vi "FGV Messwerte_FID.vi"(0 "GasValue":sgl[](array[numeric]), 1 "Messbereich":T3 items=["0-500ppm"=1, "0-2500ppm"=2, "0-10000ppm"=3], 4 "Zielmessbereich":u16, 7 "Prüfgaskonz.":sgl, 8 "Kalibrieren":T1, 9 "Aktion":T5=enum."Messen", 13 "CAL-Daten Tolernaz":T2) -> (14 "Rohwert LIN":sgl[](array[numeric]), 16 "Rohwerte":sgl[](array[numeric]), 19 "im gültigen Bereich":bool, 20 "GasValue":sgl[](array[numeric]), 21 "CAL-Daten":T4={"CH4 Null"=0.0, "CH4 Steil"=[1.0, 1.0, 1.0, 1.0], "THC Null"=0.0, "THC Steil"=[1.0, 1.0, 1.0, 1.0], "NMHC Null"=0.0, "NMHC Steil"=[1.0, 1.0, 1.0, 1.0]}, 24 "CAL-Daten Tolernaz":T2, 25 "Kalibrieren erfolgreich":bool, 27 "CAL TimeOut":bool)   [LabVIEW 2020, in "ABB-EL3000.lvlib" / "FID.lvlib" / "FID Kalibrierung.lvlib"]
uses:
  FID Kalibrierung.lvlib
  Allgemeine VI/FGV Uras26 Aktion.ctl
  Allgemeine VI/CAL-Daten FID.ctl
  Allgemeine VI/Messbereich CO lo.ctl
  Allgemeine VI/CAL-Daten Toleranz.ctl
  FID Kalibrieren.ctl
  Auto Kalibrieren/KAL Daten loggen Aktionen.ctl
  Allgemeine VI/Aktionen Cal Daten speichern.ctl
  Allgemein/allgemeine Sub-VIs.lvlib
  Allgemeine VI/Allgemeine VI.lvlib
  Auto Kalibrieren/Auto Kalibrieren.lvlib
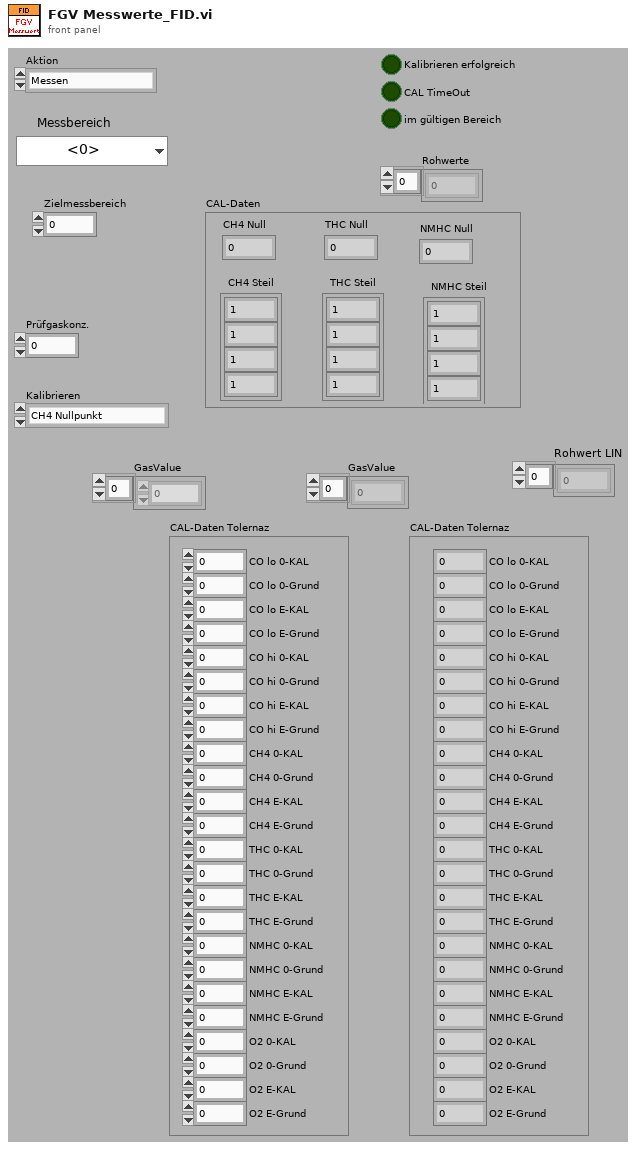
[diagram p1: front panel]
types:
  T1 = typedef "ABB-EL3000.lvlib/FID.lvlib/FID Kalibrierung.lvlib/FID Kalibrieren.ctl" = enum16{"CH4 Nullpunkt", "THC Nullpunkt", "NMHC Nullpunkt", "CH4 Endpunkt", "THC Endpunkt", "NMHC Endpunkt"}
  T2 = typedef "ABB-EL3000.lvlib/Allgemeine VI.lvlib/CAL-Daten Toleranz.ctl" = cluster{"CO lo 0-KAL":sgl, "CO lo 0-Grund":sgl, "CO lo E-KAL":sgl, "CO lo E-Grund":sgl, "CO hi 0-KAL":sgl, "CO hi 0-Grund":sgl, "CO hi E-KAL":sgl, "CO hi E-Grund":sgl, "CH4 0-KAL":sgl, "CH4 0-Grund":sgl, "CH4 E-KAL":sgl, "CH4 E-Grund":sgl, "THC 0-KAL":sgl, "THC 0-Grund":sgl, "THC E-KAL":sgl, "THC E-Grund":sgl, "NMHC 0-KAL":sgl, "NMHC 0-Grund":sgl, "NMHC E-KAL":sgl, "NMHC E-Grund":sgl, "O2 0-KAL":sgl, "O2 0-Grund":sgl, "O2 E-KAL":sgl, "O2 E-Grund":sgl}
  T3 = typedef "ABB-EL3000.lvlib/Allgemeine VI.lvlib/Messbereich CO lo.ctl" = u16
  T4 = typedef "ABB-EL3000.lvlib/Allgemeine VI.lvlib/CAL-Daten FID.ctl" = cluster{"CH4 Null":sgl, "CH4 Steil":sgl[], "THC Null":sgl, "THC Steil":sgl[], "NMHC Null":sgl, "NMHC Steil":sgl[]}
  T5 = typedef "ABB-EL3000.lvlib/Allgemeine VI.lvlib/FGV Uras26 Aktion.ctl" = enum16{"lesen", "CAL-Daten laden", "Messen", "Kalibrieren vorbereiten", "Kalibrieren", "CAL-Daten speichern", "Toleranz schreiben", "CAL-Daten kopieren"}
  T6 = typedef "Auto Kalibrieren.lvlib/KAL Daten loggen Aktionen.ctl" = enum16{"lesen", "initialisieren", "loggen"}
  T7 = typedef "ABB-EL3000.lvlib/Allgemeine VI.lvlib/Aktionen Cal Daten speichern.ctl" = enum16{"Cal Daten", "Toleranzen", "PMA", "FID", "Cal Daten PMA", "Cal Daten FID"}
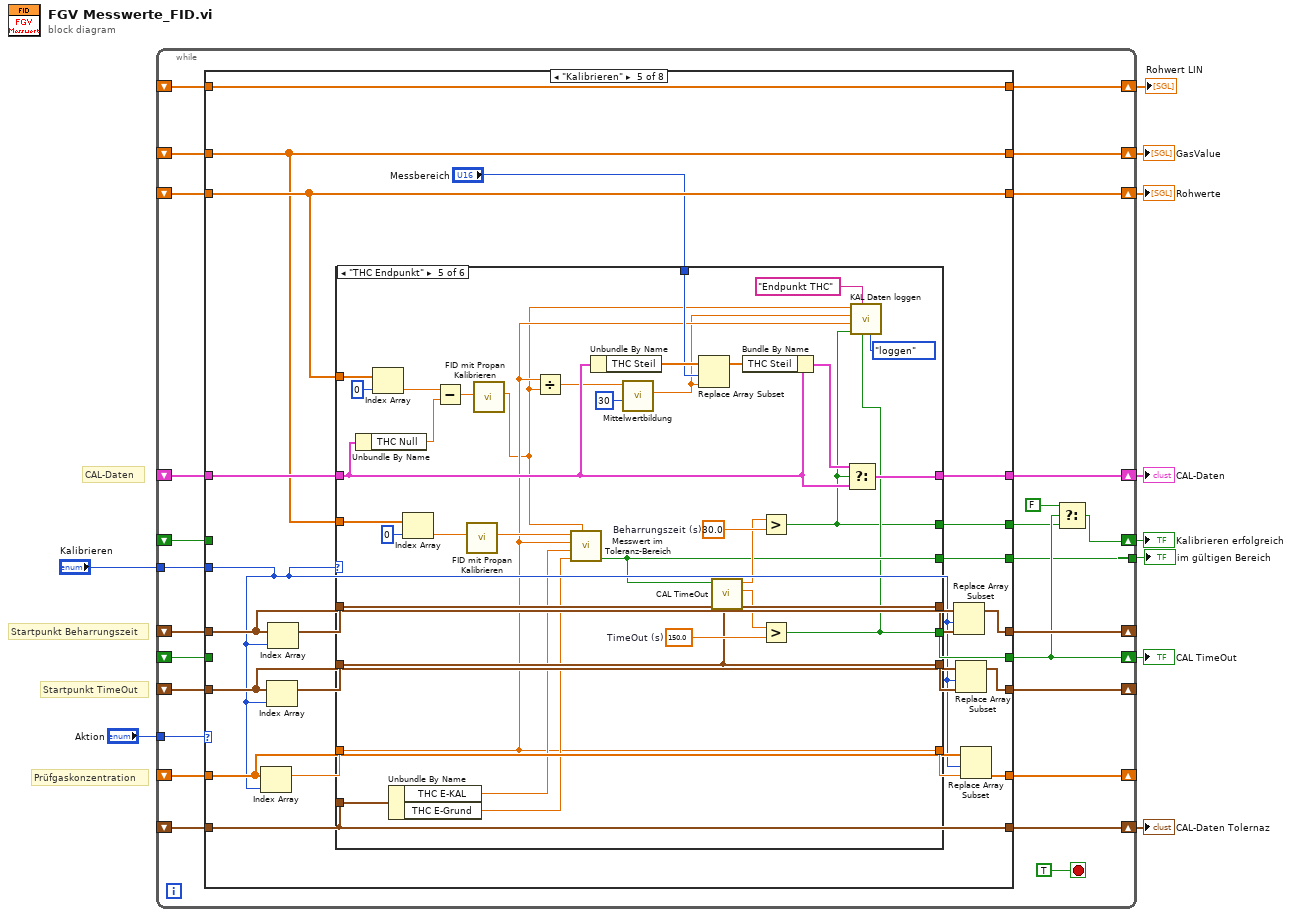
[diagram p0: block diagram]
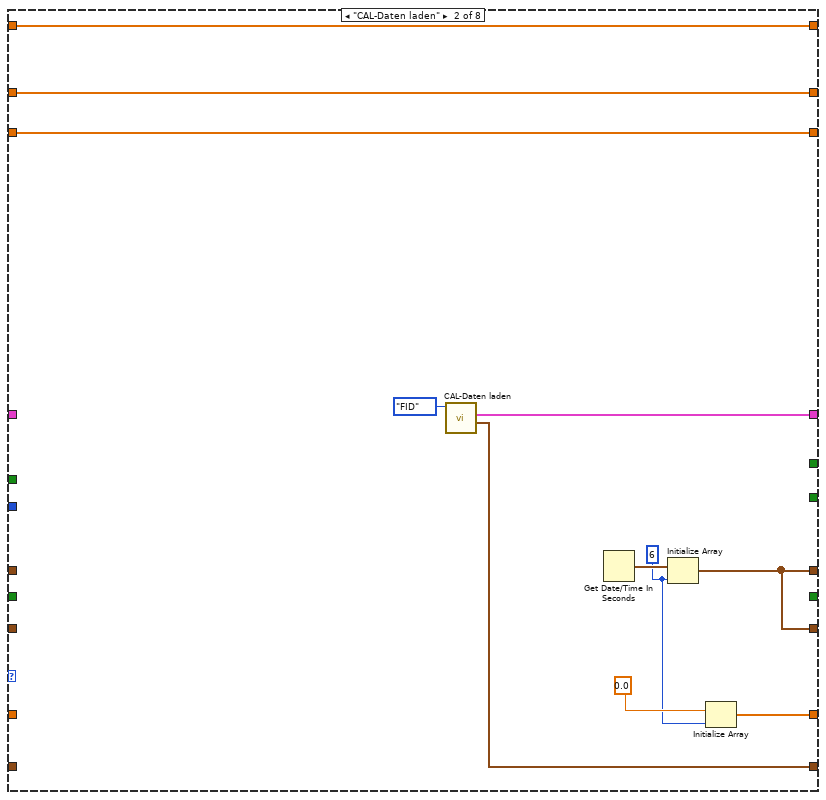
[diagram p3: hidden frame]
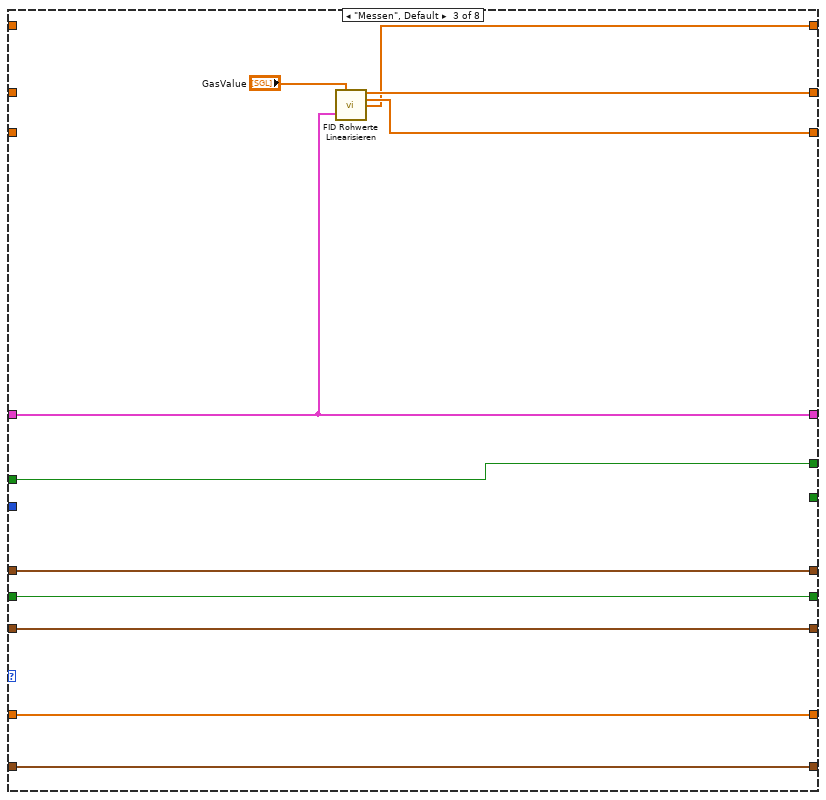
[diagram p4: hidden frame]
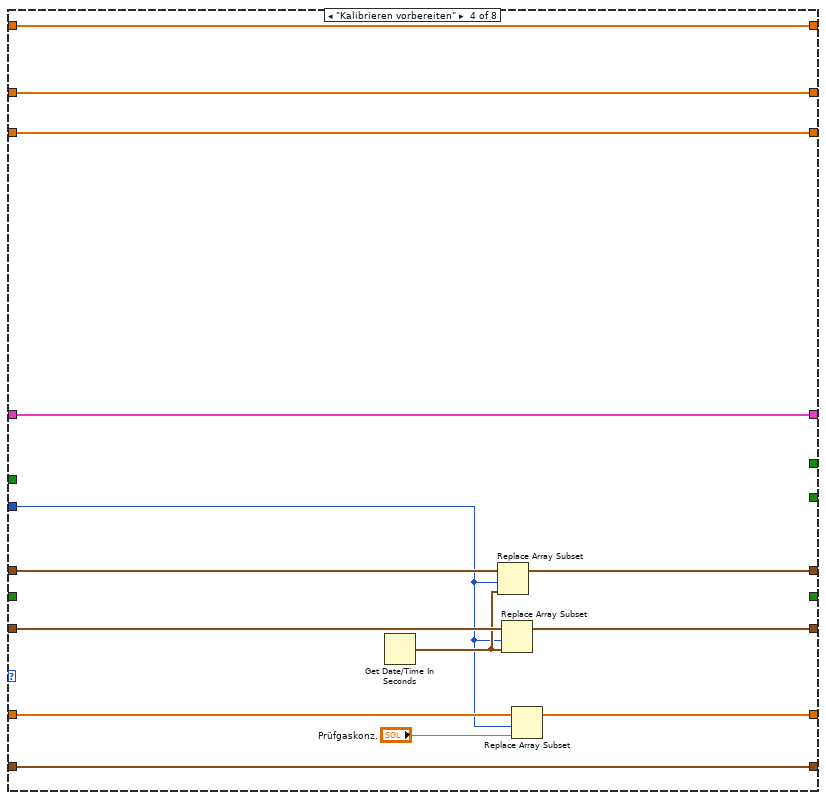
[diagram p5: hidden frame]
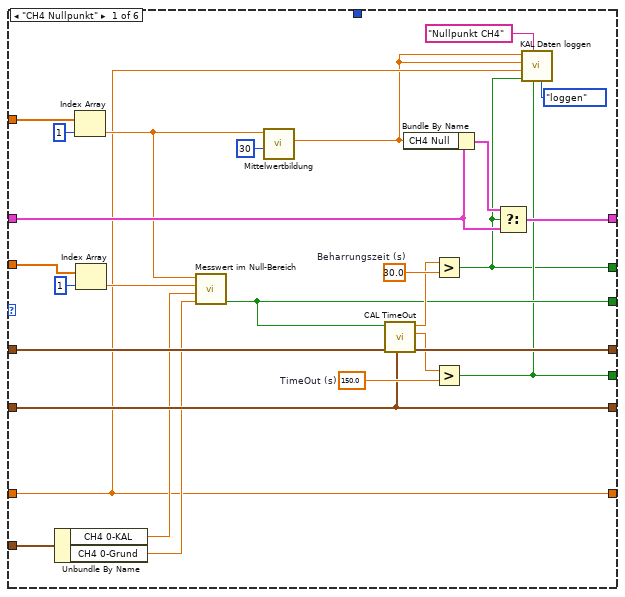
[diagram p6: hidden frame]
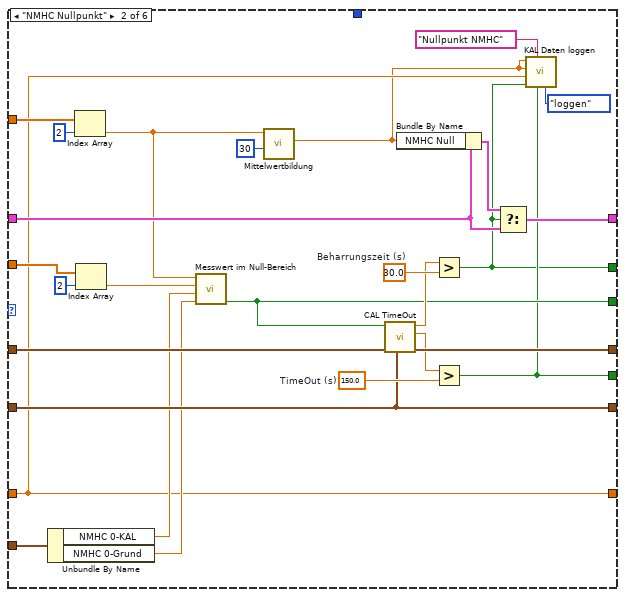
[diagram p7: hidden frame]
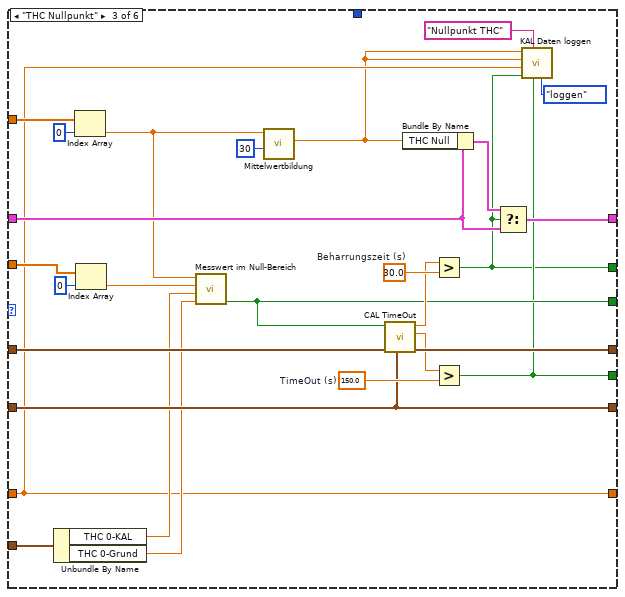
[diagram p8: hidden frame]
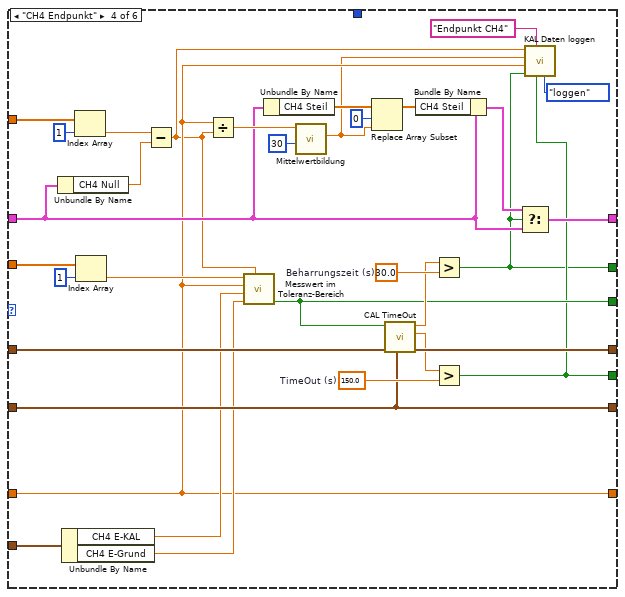
[diagram p9: hidden frame]
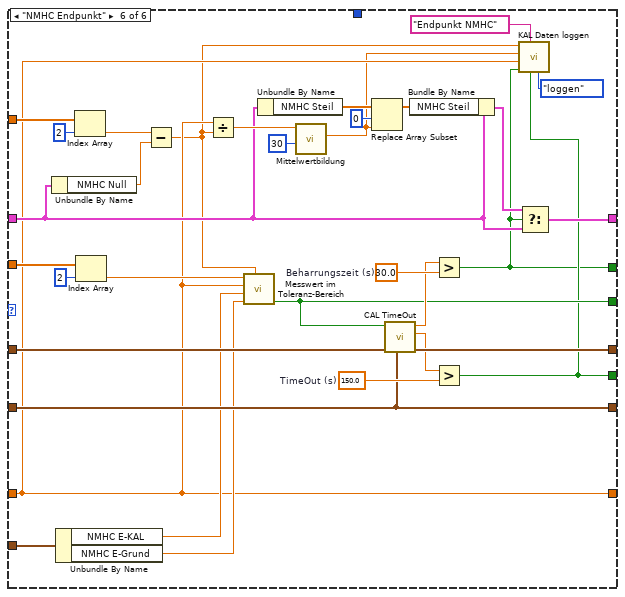
[diagram p10: hidden frame]
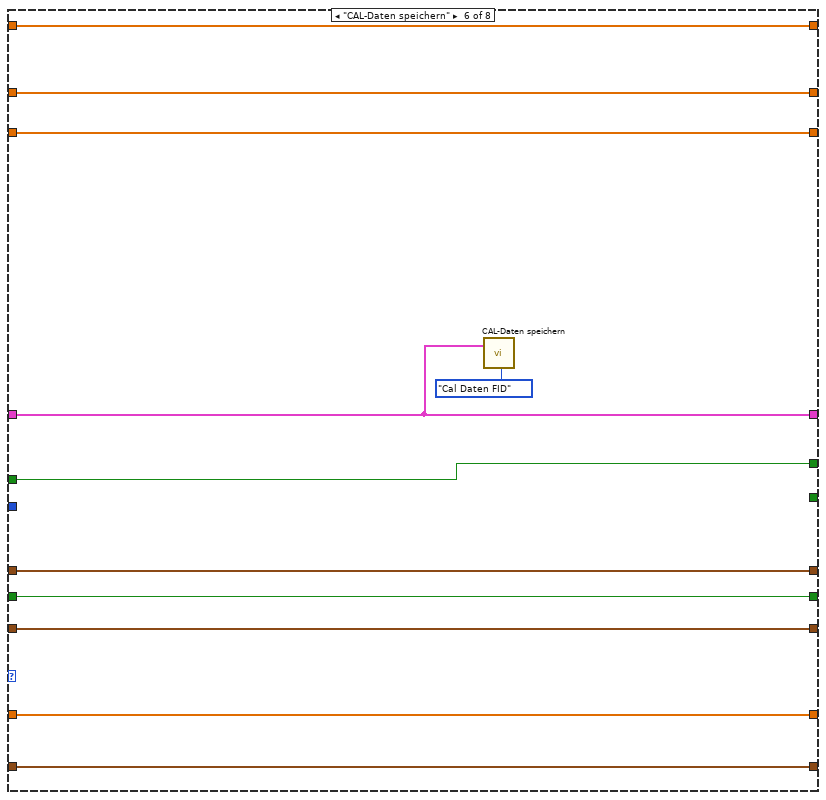
[diagram p11: hidden frame]
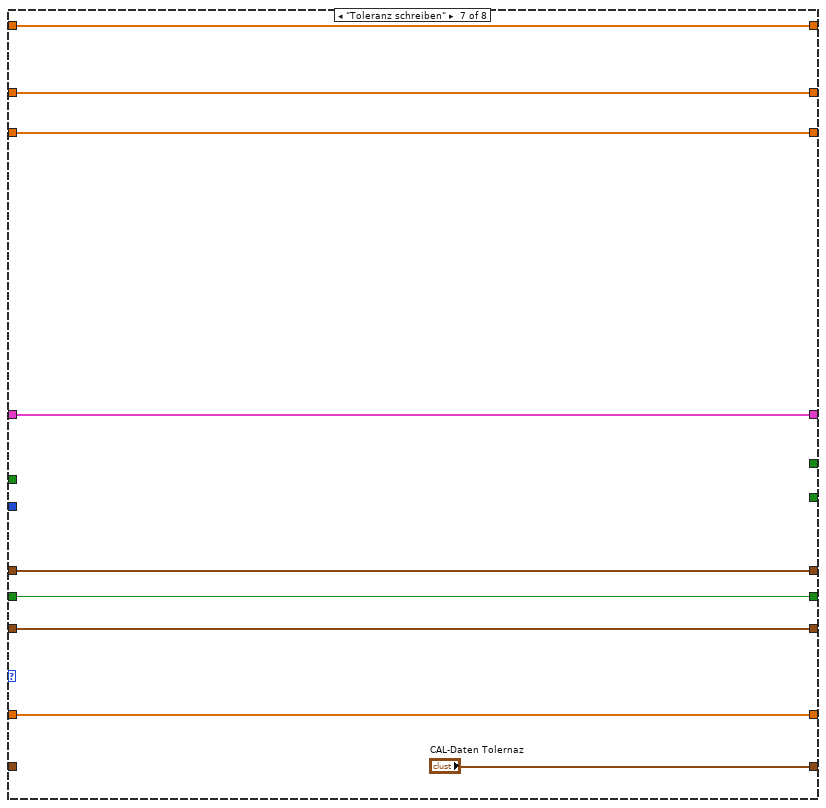
[diagram p12: hidden frame]
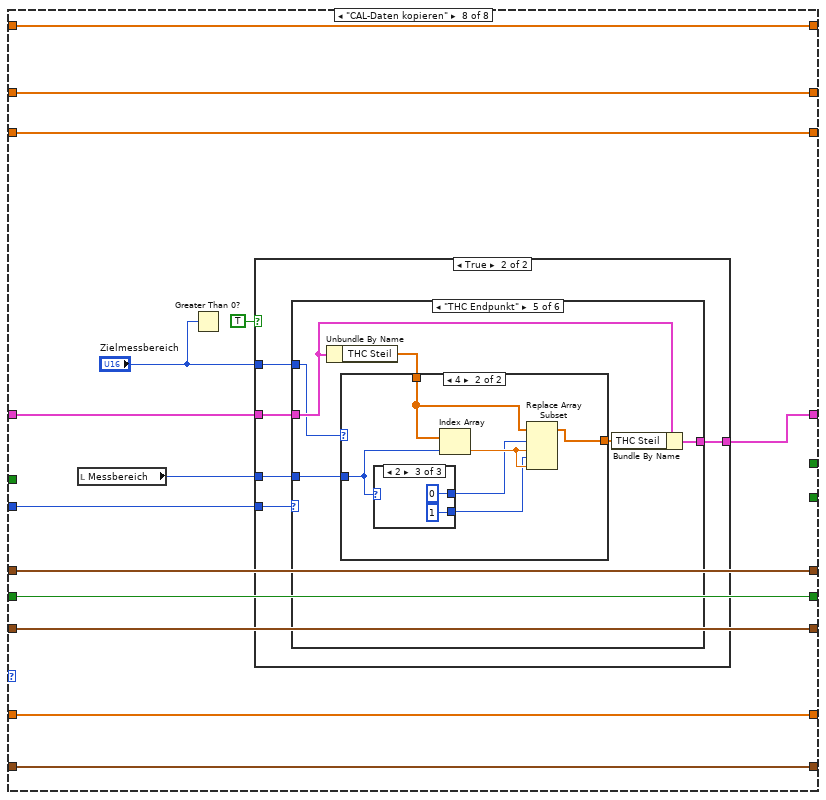
[diagram p13: hidden frame]
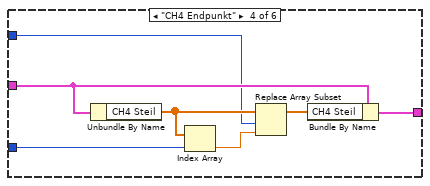
[diagram p18: hidden frame]
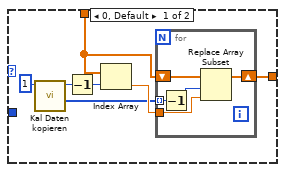
[diagram p19: hidden frame]
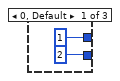
[diagram p20: hidden frame]
diagram:
  # "Prüfgaskonzentration"
  # "Startpunkt TimeOut"
  # "Startpunkt Beharrungszeit"
  # "CAL-Daten"
  n1 = while {
    tunnel: "Aktion" -> [w28]
    shift-right: [w35] -> w7
    shift-left: _ -> [w27]
    tunnel: "Kalibrieren" -> [w34]
    shift-right: [w32] -> _
    shift-left: _ -> [w31]
    shift-right: [w30] -> _
    shift-left: _ -> [w29]
    shift-right: [w22] -> w6
    shift-left: _ -> [w21]
    shift-right: [w24] -> w8
    shift-left: _ -> [w19]
    shift-right: [w26] -> w9
    shift-left: _ -> [w20]
    shift-right: [w18] -> _
    shift-left: _ -> [w33]
    shift-right: [w17] -> w5
    shift-left: _ -> [w16]
    shift-right: [w15] -> w4
    shift-left: _ -> [w14]
    tunnel: [w13] -> w3
    shift-right: [w12] -> w1
    shift-left: _ -> [w11]
    stop <- TRUE stop-if-true
    n2 = case shown="\"Kalibrieren\"" w28 {
      tunnel: w27 -> [w44 _ w62 w80 w101 w288 w304 w317]
      tunnel: [w44 w47 w62 w80 w104 w288 w304 w316] -> w35
      tunnel: w34 -> [_ _ _ w71 w84 _ _ w318]
      tunnel: w33 -> [w41 _ w63 w73 w85 w294 w301 w312]
      tunnel: [w43 w51 w67 w70 w94 w292 w303 w315] -> w32
      tunnel: w31 -> [w43 _ w67 w77 w93 w292 w303 w315]
      tunnel: [w42 w51 w66 w69 w90 w291 w302 w313] -> w30
      tunnel: w29 -> [w42 _ w66 w76 w88 w291 w302 w313]
      tunnel: [_ _ w64 _ w103 w296 w299 w314] -> w26
      tunnel: [w38 _ w65 _ w102 w295 _ _] -> w25
      tunnel: [w45 w56 w58 w81 w99 w297 w305 w319] -> w22
      tunnel: w21 -> [w45 w56 _ w81 w99 w297 w305 w319]
      tunnel: w20 -> [_ _ w64 _ _ w296 w299 w314]
      tunnel: w19 -> [w38 _ w65 _ _ w295 _ _]
      tunnel: [w41 w48 w63 w72 w86 w294 w301 w312] -> w18
      tunnel: [w40 w55 w59 w79 w98 w293 w306 w320] -> w17
      tunnel: w16 -> [w40 w55 _ w79 w98 w293 w306 w320]
      tunnel: [w39 w54 w61 w78 w100 w290 "CAL-Daten Tolernaz" w311] -> w15
      tunnel: w14 -> [w39 _ w61 w78 w100 w290 _ w311]
      tunnel: [_ _ _ _ w97 _ _ _] -> w13
      tunnel: [w37 w46 w57 w68 w82 w287 w298 w307] -> w12
      tunnel: w11 -> [w37 w46 _ w68 w82 w287 w298 w307]
      frame "lesen" {
      }
      frame "CAL-Daten laden" {
        w49 = 6 ("Dimension")
        n3 = call "CAL-Daten laden.vi"("Aktion"=enum16{"PMA", "FID"}."FID") -> ("CAL-Daten Tolernaz"=w54:T2, "CAL-Daten FID"=w47:T4)  [unwired: 6 in, 3 out]
        n4 = Get Date/Time In Seconds() -> (seconds since 1Jan1904=w52:timestamp)
        n5 = Initialize Array(w52, w49) -> (w51:timestamp[])
        n6 = Initialize Array(sgl 0.0 ("Prüfgaskonz."), w49) -> (w48:sgl[])
      }
      frame "Messen", Default {
        n7 = call "FID Rohwerte Linearisieren.vi"("GasValue"="GasValue", "CAL-Daten"=w62) -> ("Messwerte"=w59:sgl[], "Rohwert"=w58:sgl[], "Rohwert LIN"=w57:sgl[])  [unwired: 11 in]
      }
      frame "Kalibrieren vorbereiten" {
        n8 = Get Date/Time In Seconds() -> (seconds since 1Jan1904=w75:timestamp)
        n9 = Replace Array Subset(array=w77, new element=w75, index=w71) -> (w70:timestamp[])
        n10 = Replace Array Subset(array=w76, new element=w75, index=w71) -> (w69:timestamp[])
        n11 = Replace Array Subset(array=w73, new element="Prüfgaskonz.", index=w71) -> (w72:sgl[])
      }
      frame "Kalibrieren" {
        n12 = Index Array(array=w85, index=w84) -> (element=w87:sgl)
        n13 = Index Array(array=w88, index=w84) -> (element=w91:timestamp)
        n14 = Index Array(array=w93, index=w84) -> (element=w95:timestamp)
        n15 = case shown="\"THC Endpunkt\"" w84 {
          tunnel: w101 -> [w122 w149 w176 w199 w236 w267]
          tunnel: [w125 w152 w179 w212 w247 w280] -> w104
          tunnel: w87 -> [w106 w133 w160 w188 w221 w257]
          tunnel: w95 -> [w129 w156 w183 w216 w251 w284]
          tunnel: [w127 w154 w181 w214 w249 w282] -> w92
          tunnel: [w128 w155 w182 w215 w250 w283] -> w89
          tunnel: w91 -> [w128 w155 w182 w215 w250 w283]
          tunnel: [w108 w135 w162 w191 w223 w259] -> w103
          tunnel: [w107 w134 w161 w190 w222 w258] -> w102
          tunnel: [w106 w133 w160 w188 w221 w257] -> w96
          tunnel: w100 -> [w120 w147 w174 w206 w242 w274]
          tunnel: w99 -> [w119 w146 w173 w203 w239 w271]
          tunnel: w98 -> [w118 w145 w172 w201 w238 w269]
          tunnel: "Messbereich" -> [_ _ _ _ w226 _]
          tunnel: [w117 w141 w168 w200 w237 w268] -> w97
          frame "CH4 Nullpunkt" {
            w130 = sgl 150.0  # TimeOut (s)
            w131 = sgl 30.0  # Beharrungszeit (s)
            n16 = Unbundle By Name(w120) -> ("CH4 0-KAL"=w114:sgl, "CH4 0-Grund"=w113:sgl)
            n17 = Index Array(array=w119, index=1 ("Index")) -> (element=w116:sgl)
            n18 = Index Array(array=w118, index=1 ("Index")) -> (element=w115:sgl)
            n19 = call "Messwert im Null-Bereich.vi"("Toleranz Grundkalibrierung"=w113, "Toleranz letzte KAL"=w114, "Messwert"=w115, "Rohwert"=w116) -> ("im Bereich"=w117:bool)  [unwired: 7 in]
            n20 = call "Mittelwertbildung.vi"("Anzahl Werte"=u8 30, "Neuer Wert"=w116) -> ("gemittelter Wert"=w105:sgl)  [unwired: 7 in, 2 out]
            n21 = call "CAL TimeOut.vi"("CAL-Start"=w128, "im Bereich seit"=w129, "im Bereich"=w117) -> ("im Bereich seit (Ausgang)"=w127:timestamp, "Sekunden seit CAL-Start"=w126:sgl, "Sekunden im Bereich"=w124:sgl)  [unwired: 5 in]
            n22 = Bundle By Name(cluster=w122, "CH4 Null"=w105) -> (w123:T4)
            n23 = Greater?(x=w124, y=w131) -> (0:w107:bool)
            n24 = Greater?(x=w126, y=w130) -> (0:w108:bool)
            n25 = Select(t=w123, s=w107, f=w122) -> (s? t:f=w125:T4)
            n26 = call "KAL Daten loggen.vi"("Aktionen MFC loggen"=KAL_Daten_loggen_Aktionen."loggen", "TimeOUT"=w108, "Komponente"="Nullpunkt CH4", "Kalibrieren Erfolgreich"=w107, "Prüfgaskonzentration"=w106, "Kalibrierwert"=w105, "Rohwert"=w105) -> ()  [unwired: 4 in, 1 out]
          }
          frame "NMHC Nullpunkt" {
            w157 = sgl 150.0  # TimeOut (s)
            w158 = sgl 30.0  # Beharrungszeit (s)
            n27 = Unbundle By Name(w147) -> ("NMHC 0-KAL"=w143:sgl, "NMHC 0-Grund"=w142:sgl)
            n28 = Index Array(array=w146, index=2 ("Index")) -> (element=w140:sgl)
            n29 = Index Array(array=w145, index=2 ("Index")) -> (element=w144:sgl)
            n30 = call "Messwert im Null-Bereich.vi"("Toleranz Grundkalibrierung"=w142, "Toleranz letzte KAL"=w143, "Messwert"=w144, "Rohwert"=w140) -> ("im Bereich"=w141:bool)  [unwired: 7 in]
            n31 = call "Mittelwertbildung.vi"("Anzahl Werte"=u8 30, "Neuer Wert"=w140) -> ("gemittelter Wert"=w132:sgl)  [unwired: 7 in, 2 out]
            n32 = call "CAL TimeOut.vi"("CAL-Start"=w155, "im Bereich seit"=w156, "im Bereich"=w141) -> ("im Bereich seit (Ausgang)"=w154:timestamp, "Sekunden seit CAL-Start"=w153:sgl, "Sekunden im Bereich"=w151:sgl)  [unwired: 5 in]
            n33 = Bundle By Name(cluster=w149, "NMHC Null"=w132) -> (w150:T4)
            n34 = Greater?(x=w151, y=w158) -> (0:w134:bool)
            n35 = Greater?(x=w153, y=w157) -> (0:w135:bool)
            n36 = Select(t=w150, s=w134, f=w149) -> (s? t:f=w152:T4)
            n37 = call "KAL Daten loggen.vi"("Aktionen MFC loggen"=KAL_Daten_loggen_Aktionen."loggen", "TimeOUT"=w135, "Komponente"="Nullpunkt NMHC", "Kalibrieren Erfolgreich"=w134, "Prüfgaskonzentration"=w133, "Kalibrierwert"=w132, "Rohwert"=w132) -> ()  [unwired: 4 in, 1 out]
          }
          frame "THC Nullpunkt" {
            w184 = sgl 150.0  # TimeOut (s)
            w185 = sgl 30.0  # Beharrungszeit (s)
            n38 = Unbundle By Name(w174) -> ("THC 0-KAL"=w170:sgl, "THC 0-Grund"=w169:sgl)
            n39 = Index Array(array=w173, index=0 ("Index")) -> (element=w167:sgl)
            n40 = Index Array(array=w172, index=0 ("Index")) -> (element=w171:sgl)
            n41 = call "Messwert im Null-Bereich.vi"("Toleranz Grundkalibrierung"=w169, "Toleranz letzte KAL"=w170, "Messwert"=w171, "Rohwert"=w167) -> ("im Bereich"=w168:bool)  [unwired: 7 in]
            n42 = call "Mittelwertbildung.vi"("Anzahl Werte"=u8 30, "Neuer Wert"=w167) -> ("gemittelter Wert"=w159:sgl)  [unwired: 7 in, 2 out]
            n43 = call "CAL TimeOut.vi"("CAL-Start"=w182, "im Bereich seit"=w183, "im Bereich"=w168) -> ("im Bereich seit (Ausgang)"=w181:timestamp, "Sekunden seit CAL-Start"=w180:sgl, "Sekunden im Bereich"=w178:sgl)  [unwired: 5 in]
            n44 = Bundle By Name(cluster=w176, "THC Null"=w159) -> (w177:T4)
            n45 = Greater?(x=w178, y=w185) -> (0:w161:bool)
            n46 = Greater?(x=w180, y=w184) -> (0:w162:bool)
            n47 = Select(t=w177, s=w161, f=w176) -> (s? t:f=w179:T4)
            n48 = call "KAL Daten loggen.vi"("Aktionen MFC loggen"=KAL_Daten_loggen_Aktionen."loggen", "TimeOUT"=w162, "Komponente"="Nullpunkt THC", "Kalibrieren Erfolgreich"=w161, "Prüfgaskonzentration"=w160, "Kalibrierwert"=w159, "Rohwert"=w159) -> ()  [unwired: 4 in, 1 out]
          }
          frame "CH4 Endpunkt" {
            w217 = sgl 150.0  # TimeOut (s)
            w218 = sgl 30.0  # Beharrungszeit (s)
            n49 = Unbundle By Name(w199) -> ("CH4 Null"=w197:sgl)
            n50 = Unbundle By Name(w206) -> ("CH4 E-KAL"=w205:sgl, "CH4 E-Grund"=w204:sgl)
            n51 = Index Array(array=w203, index=1 ("Index")) -> (element=w198:sgl)
            n52 = Index Array(array=w201, index=1 ("Index")) -> (element=w202:sgl)
            n53 = Subtract(x=w198, y=w197) -> (x-y=w186:sgl)
            n54 = Divide(x=w188, y=w186) -> (x/y=w207:sgl)
            n55 = call "Messwert im Toleranz-Bereich.vi"("Rohwert"=w186, "Toleranz Grundkalibrierung"=w204, "Toleranz in % letzte KAL"=w205, "Prüfgas-Konzentration"=w188, "Messwert"=w202) -> ("im Bereich"=w200:bool)  [unwired: 6 in]
            n56 = Unbundle By Name(w199) -> ("CH4 Steil"=w210:sgl[])
            n57 = call "Mittelwertbildung.vi"("Anzahl Werte"=u8 30, "Neuer Wert"=w207) -> ("gemittelter Wert"=w187:sgl)  [unwired: 7 in, 2 out]
            n58 = Replace Array Subset(array=w210, new element=w187, index=0 ("Index")) -> (w209:sgl[])
            n59 = call "CAL TimeOut.vi"("CAL-Start"=w215, "im Bereich seit"=w216, "im Bereich"=w200) -> ("im Bereich seit (Ausgang)"=w214:timestamp, "Sekunden seit CAL-Start"=w213:sgl, "Sekunden im Bereich"=w211:sgl)  [unwired: 5 in]
            n60 = Bundle By Name(cluster=w199, "CH4 Steil"=w209) -> (w196:T4)
            n61 = Greater?(x=w211, y=w218) -> (0:w190:bool)
            n62 = Greater?(x=w213, y=w217) -> (0:w191:bool)
            n63 = Select(t=w196, s=w190, f=w199) -> (s? t:f=w212:T4)
            n64 = call "KAL Daten loggen.vi"("Aktionen MFC loggen"=KAL_Daten_loggen_Aktionen."loggen", "TimeOUT"=w191, "Komponente"="Endpunkt CH4", "Kalibrieren Erfolgreich"=w190, "Prüfgaskonzentration"=w188, "Kalibrierwert"=w187, "Rohwert"=w186) -> ()  [unwired: 4 in, 1 out]
          }
          frame "THC Endpunkt" {
            w252 = sgl 150.0  # TimeOut (s)
            w253 = sgl 30.0  # Beharrungszeit (s)
            n65 = Unbundle By Name(w236) -> ("THC Null"=w231:sgl)
            n66 = Index Array(array=w239, index=0 ("Index")) -> (element=w232:sgl)
            n67 = Unbundle By Name(w242) -> ("THC E-KAL"=w241:sgl, "THC E-Grund"=w240:sgl)
            n68 = Index Array(array=w238, index=0 ("Index")) -> (element=w229:sgl)
            n69 = Subtract(x=w232, y=w231) -> (x-y=w230:sgl)
            n70 = call "FID mit Propan Kalibrieren.vi"("Wert"=w229) -> ("Wert"=w228:sgl)  [unwired: 9 in, 1 out]
            n71 = call "FID mit Propan Kalibrieren.vi"("Wert"=w230) -> ("Wert"=w220:sgl)  [unwired: 9 in, 1 out]
            n72 = Divide(x=w221, y=w220) -> (x/y=w227:sgl)
            n73 = call "Messwert im Toleranz-Bereich.vi"("Rohwert"=w220, "Toleranz Grundkalibrierung"=w240, "Toleranz in % letzte KAL"=w241, "Prüfgas-Konzentration"=w221, "Messwert"=w228) -> ("im Bereich"=w237:bool)  [unwired: 6 in]
            n74 = Unbundle By Name(w236) -> ("THC Steil"=w245:sgl[])
            n75 = call "Mittelwertbildung.vi"("Anzahl Werte"=u8 30, "Neuer Wert"=w227) -> ("gemittelter Wert"=w219:sgl)  [unwired: 7 in, 2 out]
            n76 = Replace Array Subset(array=w245, new element=w219, index=w226) -> (w244:sgl[])
            n77 = call "CAL TimeOut.vi"("CAL-Start"=w250, "im Bereich seit"=w251, "im Bereich"=w237) -> ("im Bereich seit (Ausgang)"=w249:timestamp, "Sekunden seit CAL-Start"=w248:sgl, "Sekunden im Bereich"=w246:sgl)  [unwired: 5 in]
            n78 = Bundle By Name(cluster=w236, "THC Steil"=w244) -> (w235:T4)
            n79 = Greater?(x=w246, y=w253) -> (0:w222:bool)
            n80 = Greater?(x=w248, y=w252) -> (0:w223:bool)
            n81 = Select(t=w235, s=w222, f=w236) -> (s? t:f=w247:T4)
            n82 = call "KAL Daten loggen.vi"("Aktionen MFC loggen"=KAL_Daten_loggen_Aktionen."loggen", "TimeOUT"=w223, "Komponente"="Endpunkt THC", "Kalibrieren Erfolgreich"=w222, "Prüfgaskonzentration"=w221, "Kalibrierwert"=w219, "Rohwert"=w220) -> ()  [unwired: 4 in, 1 out]
          }
          frame "NMHC Endpunkt" {
            w285 = sgl 150.0  # TimeOut (s)
            w286 = sgl 30.0  # Beharrungszeit (s)
            n83 = Unbundle By Name(w267) -> ("NMHC Null"=w265:sgl)
            n84 = Unbundle By Name(w274) -> ("NMHC E-KAL"=w273:sgl, "NMHC E-Grund"=w272:sgl)
            n85 = Index Array(array=w271, index=2 ("Index")) -> (element=w266:sgl)
            n86 = Index Array(array=w269, index=2 ("Index")) -> (element=w270:sgl)
            n87 = Subtract(x=w266, y=w265) -> (x-y=w255:sgl)
            n88 = Divide(x=w257, y=w255) -> (x/y=w275:sgl)
            n89 = call "Messwert im Toleranz-Bereich.vi"("Rohwert"=w255, "Toleranz Grundkalibrierung"=w272, "Toleranz in % letzte KAL"=w273, "Prüfgas-Konzentration"=w257, "Messwert"=w270) -> ("im Bereich"=w268:bool)  [unwired: 6 in]
            n90 = Unbundle By Name(w267) -> ("NMHC Steil"=w278:sgl[])
            n91 = call "Mittelwertbildung.vi"("Anzahl Werte"=u8 30, "Neuer Wert"=w275) -> ("gemittelter Wert"=w256:sgl)  [unwired: 7 in, 2 out]
            n92 = Replace Array Subset(array=w278, new element=w256, index=0 ("Index")) -> (w277:sgl[])
            n93 = call "CAL TimeOut.vi"("CAL-Start"=w283, "im Bereich seit"=w284, "im Bereich"=w268) -> ("im Bereich seit (Ausgang)"=w282:timestamp, "Sekunden seit CAL-Start"=w281:sgl, "Sekunden im Bereich"=w279:sgl)  [unwired: 5 in]
            n94 = Bundle By Name(cluster=w267, "NMHC Steil"=w277) -> (w264:T4)
            n95 = Greater?(x=w279, y=w286) -> (0:w258:bool)
            n96 = Greater?(x=w281, y=w285) -> (0:w259:bool)
            n97 = call "KAL Daten loggen.vi"("Aktionen MFC loggen"=KAL_Daten_loggen_Aktionen."loggen", "TimeOUT"=w259, "Komponente"="Endpunkt NMHC", "Kalibrieren Erfolgreich"=w258, "Prüfgaskonzentration"=w257, "Kalibrierwert"=w256, "Rohwert"=w255) -> ()  [unwired: 4 in, 1 out]
            n98 = Select(t=w264, s=w258, f=w267) -> (s? t:f=w280:T4)
          }
        }
        n99 = Replace Array Subset(array=w93, new element=w92, index=w84) -> (w94:timestamp[])
        n100 = Replace Array Subset(array=w88, new element=w89, index=w84) -> (w90:timestamp[])
        n101 = Replace Array Subset(array=w85, new element=w96, index=w84) -> (w86:sgl[])
      }
      frame "CAL-Daten speichern" {
        n102 = call "CAL-Daten speichern.vi"("CAL-Daten FID"=w288, "Aktionen Kal Daten speichern"=Aktionen_Cal_Daten_speichern."Cal Daten FID") -> ()  [unwired: 18 in]
      }
      frame "Toleranz schreiben" {
      }
      frame "CAL-Daten kopieren" {
        n103 = local read "Messbereich"() -> (w309:T3)
        n104 = Greater Than 0?(x="Zielmessbereich") -> ()  [unwired: 1 out]
        n105 = case shown="True" TRUE {
          tunnel: w318 -> [_ w326]
          tunnel: w317 -> [w321 w325]
          tunnel: w309 -> [_ w324]
          tunnel: [w321 w323] -> w316
          tunnel: "Zielmessbereich" -> [_ w322]
          frame False {
          }
          frame True {
            n106 = case shown="\"THC Endpunkt\"" w326 {
              tunnel: w325 -> [w327 w328 w329 w335 w341 w372]
              tunnel: w324 -> [_ _ _ w333 w339 w370]
              tunnel: w322 -> [_ _ _ w331 w337 w368]
              tunnel: [w327 w328 w329 w330 w338 w367] -> w323
              frame "CH4 Nullpunkt", Default {
              }
              frame "THC Nullpunkt" {
              }
              frame "NMHC Nullpunkt" {
              }
              frame "CH4 Endpunkt" {
                n107 = Unbundle By Name(w335) -> ("CH4 Steil"=w334:sgl[])
                n108 = Index Array(array=w334, index=w333) -> (element=w332:sgl)
                n109 = Replace Array Subset(array=w334, new element=w332, index=w331) -> (w336:sgl[])
                n110 = Bundle By Name(cluster=w335, "CH4 Steil"=w336) -> (w330:T4)
              }
              frame "THC Endpunkt" {
                n111 = Unbundle By Name(w341) -> ("THC Steil"=w340:sgl[])
                n112 = case shown="4" w337 {
                  tunnel: [w349 w357] -> w342
                  tunnel: w340 -> [w348 w360]
                  tunnel: w339 -> [_ w359]
                  frame 0, Default {
                    n113 = call "Kal Daten kopieren.vi"("Komponente"=1) -> ("Ziel MB"=w344:i32[], "Kalibrierter MB"=w346:i32)  [unwired: 9 in]
                    n114 = Decrement(x=w346) -> (x-1=w343:i32)
                    n115 = Index Array(array=w348, index=w343) -> (element=w347:sgl)
                    n116 = for {
                      tunnel: w347 -> [w352]
                      shift-right: [w354] -> w349
                      shift-left: w348 -> [w353]
                      tunnel: w344 -> [w351] mode=indexing
                      n117 = Decrement(x=w351) -> (x-1=w350:i32)
                      n118 = Replace Array Subset(array=w353, new element=w352, index=w350) -> (w354:sgl[])
                    }
                  }
                  frame 4 {
                    n119 = case shown="2" w359 {
                      tunnel: [1 ("Index") 0 ("Index") 0 ("Index")] -> w356
                      tunnel: [2 ("Index") 2 ("Index") 1 ("Index")] -> w355
                      frame 0, Default {
                      }
                      frame 1 {
                      }
                      frame 2 {
                      }
                    }
                    n120 = Index Array(array=w360, index=w359) -> (element=w358:sgl)
                    n121 = Replace Array Subset(array=w360, new element #1=w358, index #1=w356, new element #2=w358, index #2=w355) -> (w357:sgl[])
                  }
                }
                n122 = Bundle By Name(cluster=w341, "THC Steil"=w342) -> (w338:T4)
              }
              frame "NMHC Endpunkt" {
                n123 = Unbundle By Name(w372) -> ("NMHC Steil"=w371:sgl[])
                n124 = Index Array(array=w371, index=w370) -> (element=w369:sgl)
                n125 = Replace Array Subset(array=w371, new element=w369, index=w368) -> (w373:sgl[])
                n126 = Bundle By Name(cluster=w372, "NMHC Steil"=w373) -> (w367:T4)
              }
            }
          }
        }
      }
    }
    n127 = Select(t=FALSE, s=w26, f=w25) -> (s? t:f=w24:bool)
  }
  "Kalibrieren erfolgreich" <- w8
  "CAL TimeOut" <- w9
  "CAL-Daten" <- w7
  "Rohwerte" <- w6
  "GasValue" <- w5
  "CAL-Daten Tolernaz" <- w4
  "im gültigen Bereich" <- w3
  "Rohwert LIN" <- w1
